vi "Get_MES_Path.vi"() -> (2 "路径":path, 3 "value":string)   [LabVIEW 2018]
uses:
  Global.vi
  <vilib>/Utility/config.llb/Read Key (String).vi
  <vilib>/Utility/config.llb/NI_LVConfig.lvlib
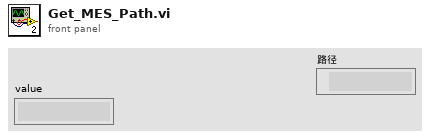
[diagram p1: front panel]
types:
  T1 = typedef "NI_LVConfig.lvlib/Config Data RefNum.ctl" = refnum<k1>
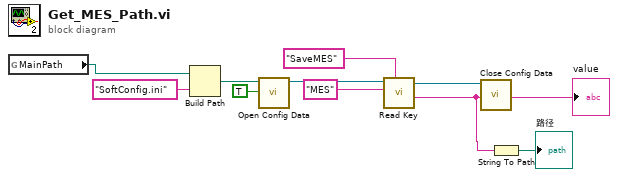
[diagram p0: block diagram]
diagram:
  n1 = global read "Global.vi" "MainPath"() -> (w4:path)
  n2 = Build Path(base path=w4, name or relative path="SoftConfig.ini" ("名称或相对路径")) -> (appended path=w5:path)
  n3 = call <vilib>:"Open Config Data.vi"("create file if necessary (T)"=TRUE, "configuration file path"=w5) -> ("refnum"=w3:T1)  [unwired: 7 in, 2 out]
  n4 = call-poly <vilib>:"Read Key.vi"("section"="SaveMES", "key"="MES", "refnum"=w3) -> ("value"=w2:string, "refnum out"=w10:T1)  [unwired: 5 in, 2 out]
  "value" <- w2
  n5 = call <vilib>:"Close Config Data.vi"("refnum"=w10) -> ()  [unwired: 9 in, 2 out]
  n6 = String To Path(string=w2) -> (path=→"路径":path)
